vi "Receive_Analogues.vi"(2 "Nr of Values":u32, 3 "Memory to Write":u8) -> (0 "Error Out":u8, 1 "Aborted":bool)   [LabVIEW 2017]
uses:
  <vilib>/rvi/interface/RandomDataEmulation/niFpgaRandomDataHandleErrors.vi
  <vilib>/rvi/Memory/Memory_Emulation/nirvimemoryFastEmulation.vi
  <vilib>/rvi/Memory/Memory_Emulation/nirvimemoryEmulation.vi
  <vilib>/rvi/Emulation/niFpgaEmulationIsFPGAContextNoSignature.vi
  <vilib>/rvi/DataTransferAndStorage/Container/Common/niFpgaContainerGetUniqueNameForEmu.vi
  <vilib>/rvi/Emulation/niFpgaProcessEmulError.vi
  <vilib>/rvi/Emulation/niFpgaSctlEmulationGetInTimedLoop.vi
  <vilib>/rvi/errors/nirviReportUnexpectedCaseInternalError (U32).vi
  <vilib>/rvi/DataTransferAndStorage/Container/XNode/niFpgaContainer.xnode
  <vilib>/rvi/interface/RandomDataEmulation/nirviRandomDataFpgaReadWriteTemplate.vi
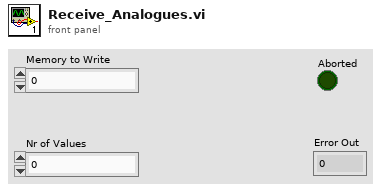
[diagram p1: front panel]
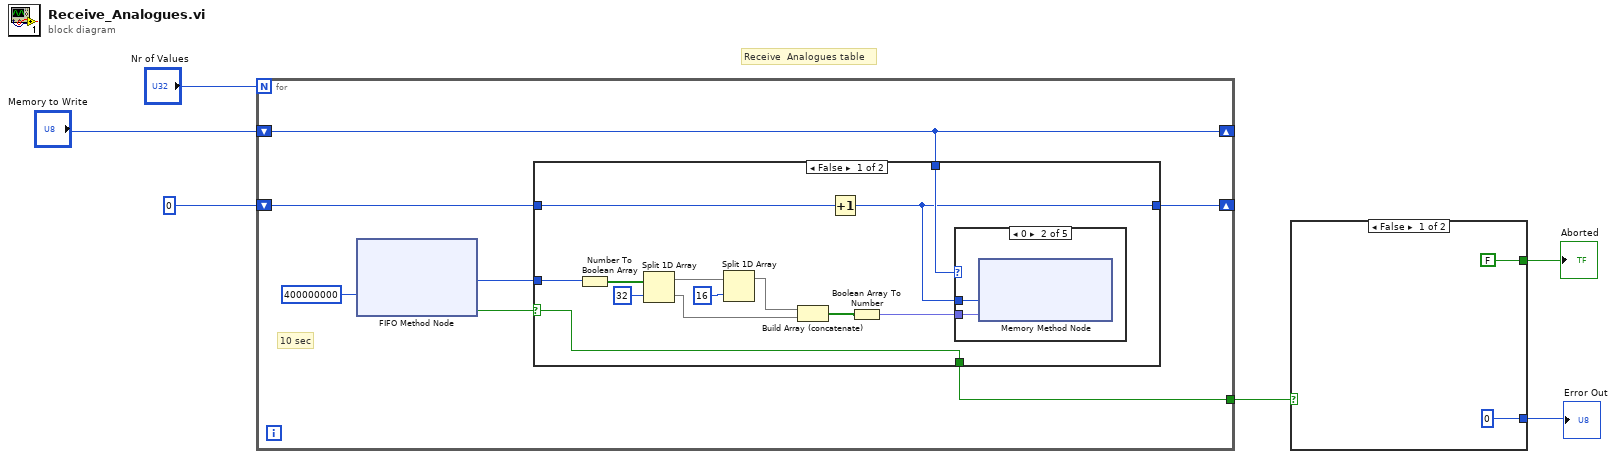
[diagram p0: block diagram]
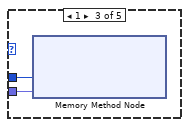
[diagram p3: hidden frame]
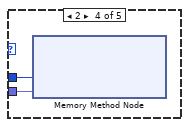
[diagram p4: hidden frame]
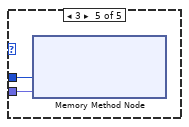
[diagram p5: hidden frame]
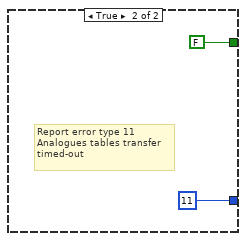
[diagram p7: hidden frame]
diagram:
  # "Receive  Analogues table"
  n1 = for {
    N: "Nr of Values" -> [_]
    shift-right: [w13] -> _
    shift-left: "Memory to Write" -> [w13]
    shift-right: [w8] -> _
    shift-left: u16 0 -> [w9]
    tunnel: [w7] -> w5
    # "10 sec"
    n2 = xnode ("FIFO Method Node")("Timeout"=400000000) -> ("Element"=w11:u64, "Timed Out?"=w10:bool)  [unwired: 1 in, 1 out]
    n3 = case shown="False" w10 {
      selector: w10 -> [w16 w36]
      tunnel: w13 -> [w26 _]
      tunnel: w11 -> [w21 _]
      tunnel: [w16 w36] -> w7
      tunnel: w9 -> [w15 w35]
      tunnel: [w14 w35] -> w8
      frame False {
        n4 = Number To Boolean Array(number=w21) -> (Boolean array=w24:bool[])
        n5 = Split 1D Array(array=w24, index=32) -> (first subarray=w23:bool[], second subarray=w18:bool[])
        n6 = Split 1D Array(array=w23, index=16) -> (first subarray=w17:bool[])  [unwired: 1 out]
        n7 = Build Array (concatenate)(w17, w18) -> (w20:bool[])
        n8 = Increment(x=w15) -> (x+1=w14:u16)
        n9 = Boolean Array To Number(Boolean array=w20) -> (number=w19:fxp<+/-,48,48>)
        n10 = case shown="0" w26 {
          tunnel: w19 -> [_ w28 w30 w32 w33]
          tunnel: w14 -> [_ w27 w29 w31 w34]
          frame 255, Default {
          }
          frame 0 {
            n11 = xnode ("Memory Method Node")("Address"=w27, "Data"=w28) -> ()  [unwired: 1 in, 1 out]
          }
          frame 1 {
            n12 = xnode ("Memory Method Node")("Address"=w29, "Data"=w30) -> ()  [unwired: 1 in, 1 out]
          }
          frame 2 {
            n13 = xnode ("Memory Method Node")("Address"=w31, "Data"=w32) -> ()  [unwired: 1 in, 1 out]
          }
          frame 3 {
            n14 = xnode ("Memory Method Node")("Address"=w34, "Data"=w33) -> ()  [unwired: 1 in, 1 out]
          }
        }
      }
      frame True {
      }
    }
  }
  n15 = case shown="False" w5 {
    tunnel: [u8 0 u8 11 ("Element")] -> w3
    tunnel: [FALSE FALSE] -> w2
    frame False {
    }
    frame True {
      # "Report error type 11\nAnalogues tables transfer \ntimed-out"
    }
  }
  "Error Out" <- w3
  "Aborted" <- w2
